vi "test Loopback_Complex_withOverflow.vi"(8 "error in":errorcluster, 11 "TestCase in":refnum<class "Single Core Complex Loopback.lvclass">) -> (0 "error out":errorcluster, 3 "TestCase out":refnum<class "Single Core Complex Loopback.lvclass">)   [LabVIEW 2020, in "Single Core Complex Loopback.lvclass"]
uses:
  Single Core Complex Loopback.lvclass
  C:/Git/niveristand-custom-device-testing-tools/VeriStandTestCase/VeriStandTestCase.lvclass
  <vilib>/numeric/Random Number (Range) DBL.vi
  <vilib>/NI VeriStand/Execution/Workspace/NI VeriStand - Set Single Channel Value.vi
  <vilib>/NI VeriStand/Execution/Workspace/NI VeriStand - Get Single Channel Value.vi
  <vilib>/addons/_JKI Toolkits/VI Tester/TestCase.llb/TestCase.lvclass
  niveristand-custom-device-testing-tools/VeriStandTestUtilities/VeriStandTestUtilities.lvlib
  <vilib>/NI VeriStand/Execution/Workspace/NI_VS Workspace ExecutionAPI.lvlib
  C:/Program Files (x86)/National Instruments/LabVIEW 2020/vi.lib/addons/_JKI Toolkits/VI Tester/TestCase.llb/TestCase.lvclass
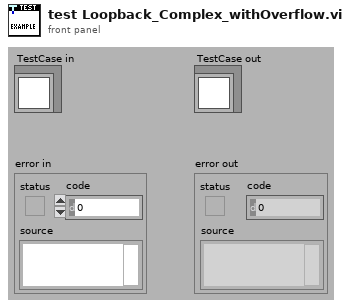
[diagram p1: front panel]
types:
  T1 = typedef "NI_VS Workspace ExecutionAPI.lvlib/WorkspaceAPI.ctl" = refnum<k24>
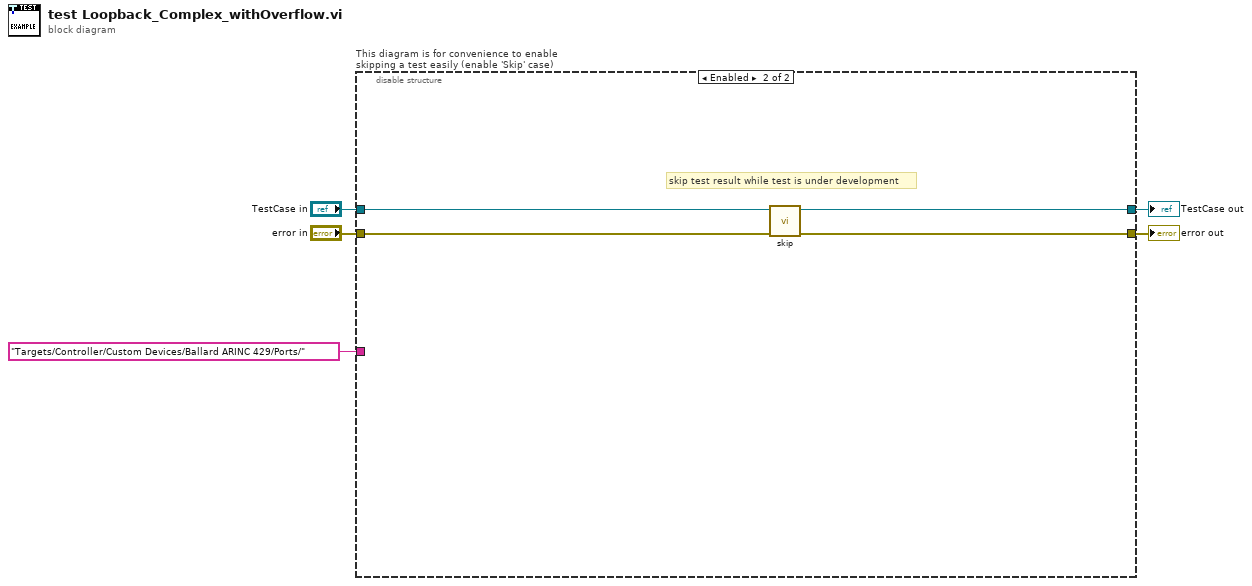
[diagram p0: block diagram]
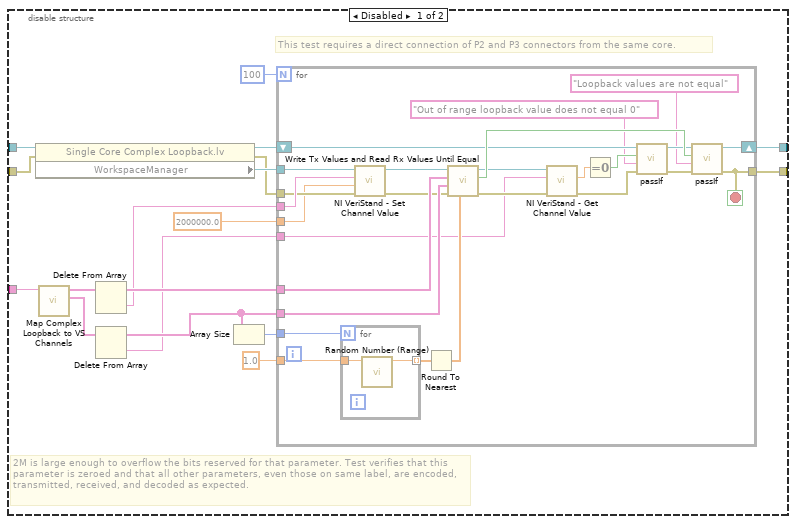
[diagram p2: hidden frame]
diagram:
  n1 = disable-structure "This diagram is for convenience to enable skipping a test easily (enable 'Skip' case)" shown="Enabled" {
    disable-tunnel: "TestCase in" -> [w10 w55]
    disable-tunnel: [w6 w53] -> w2
    disable-tunnel: [w7 w54] -> w4
    disable-tunnel: "error in" -> [w9 w52]
    disable-tunnel: "Targets/Controller/Custom Devices/Ballard ARINC 429/Ports/" ("Channel") -> [w8 _]
    frame Disabled {
      # "2M is large enough to overflow the bits reserved for that parameter. Test verifies that this parameter is zeroed and that all other parameters, even those on same label, are encoded, transmitted, received, and decoded as expected."
      # "This test requires a direct connection of P2 and P3 connectors from the same core."
      n2 = property class="Single Core Complex Loopback.lv"(reference=w10, error in=w9) -> (reference out=w21:refnum<class "Single Core Complex Loopback.lvclass">, error out=w22:errorcluster, "WorkspaceManager"=w23:T1)
      n3 = call "Map Complex Loopback to VS Channels.vi"("Base Path to Ports"=w8) -> ("Rx Channel Array"=w15:string[], "Tx Channel Array"=w16:string[])  [unwired: 9 in]
      n4 = Delete From Array(array=w16) -> (deleted portion=w12:string, array with subset deleted=w14:string[])  [unwired: 2 in]
      n5 = Delete From Array(array=w15) -> (deleted portion=w11:string, array with subset deleted=w13:string[])  [unwired: 2 in]
      n6 = Array Size(array=w13) -> (size(s)=w18:i32)
      n7 = for {
        N: 100 ("x") -> [_]
        tunnel: w14 -> [w45]
        tunnel: w23 -> [w36]
        tunnel: w22 -> [w37]
        tunnel: w13 -> [w44]
        shift-right: [w49] -> w6
        shift-left: w21 -> [w30]
        tunnel: [w48] -> w7
        tunnel: 1.0 ("upper bound (100)") -> [w46]
        tunnel: w18 -> [w41]
        tunnel: w12 -> [w40]
        tunnel: 2000000.0 ("Value") -> [w35]
        tunnel: w11 -> [w28]
        stop <- w48 stop-if-true
        n8 = for {
          N: w41 -> [_]
          tunnel: [w51] -> w47 mode=indexing
          tunnel: w46 -> [w50]
          n9 = call-poly <vilib>:"Random Number (Range).vi"("upper bound (100)"=w50) -> ("number"=w51:dbl)  [unwired: 10 in]
        }
        n10 = call-poly <vilib>:"NI VeriStand - Set Channel Value.vi"("error in (no error)"=w37, "Value"=w35, "Channel"=w40, "WorkspaceManager in"=w36) -> ("error out"=w38:errorcluster, "WorkspaceManager out"=w39:T1)  [unwired: 6 in]
        n11 = Round To Nearest(number=w47) -> (nearest integer value=w42:dbl[])
        n12 = call "Write Tx Values and Read Rx Values Until Equal.vi"("Tx values"=w42, "error in"=w38, "Rx aliases"=w44, "Tx aliases"=w45, "workspace manager in"=w39) -> ("error out"=w33:errorcluster, "values equal"=w43:bool, "workspace manager out"=w34:T1)  [unwired: 4 in]
        n13 = call-poly <vilib>:"NI VeriStand - Get Channel Value.vi"("error in (no error)"=w33, "Channel"=w28, "WorkspaceManager in"=w34) -> ("error out"=w29:errorcluster, "Value"=w32:dbl)  [unwired: 6 in, 1 out]
        n14 = Equal To 0?(x=w32) -> (x = 0?=w31:bool)
        n15 = call-dynamic "passIf.vi"("error in (no error)"=w29, "message (\"\")"="Out of range loopback value does not equal 0" ("message (\"\")"), "pass"=w31, "TestCase in"=w30) -> ("error out"=w26:errorcluster, "TestCase out"=w27:refnum<class "Single Core Complex Loopback.lvclass">)  [unwired: 6 in]
        n16 = call-dynamic "passIf.vi"("error in (no error)"=w26, "message (\"\")"="Loopback values are not equal" ("message (\"\")"), "pass"=w43, "TestCase in"=w27) -> ("error out"=w48:errorcluster, "TestCase out"=w49:refnum<class "Single Core Complex Loopback.lvclass">)  [unwired: 6 in]
      }
    }
    frame Enabled {
      # "skip test result while test is under development"
      n17 = call <vilib>:"skip.vi"("error in (no error)"=w52, "TestCase in"=w55) -> ("error out"=w54:errorcluster, "TestCase out"=w53:refnum<class "Single Core Complex Loopback.lvclass">)  [unwired: 8 in]
    }
  }
  "error out" <- w4
  "TestCase out" <- w2
